vi "RobotDriveOpen6MotorWithTalonSRX.vi"(0 "Left Motor 1":u8=20, 1 "Left Motor 2":u8=20, 2 "Left Motor 3":u8=20, 3 "Right Motor 1":u8=20, 4 "Right Motor 2":u8=20, 5 "Right Motor 3":u8=20, 7 "error in (no error)":errorcluster, 8 "Left Motor Inverted 1":bool, 9 "Right Motor Inverted 1":bool, 10 "Left Motor Inverted 2":bool, 11 "Right Motor Inverted 2":bool, 12 "Left Motor Inverted 3":bool, 13 "Right Motor Inverted 3":bool) -> (20 "RobotDriveDevRef":T1={"DevStatus"={"status"=FALSE, "code"=0, "source"=""}, "Motors[]"=[], "Square Inputs"=FALSE, "Max Output"=1.0}, 27 "error out":errorcluster)   [LabVIEW 2015]
doc: "Opens a reference to the robot drive for a four-motor robot using VictorSP motor controllers.\n\nThis software is licensed. Open the labview\\readme\\WPI Robotics Library Open Source License.txt file for more information."
uses:
  <vilib>/Rock Robotics/WPI/RobotDrive/WPI_RobotDriveDevRef.ctl
  <vilib>/Rock Robotics/WPI/MotorControl/WPI_MotorControlDeviceRef.ctl
  <vilib>/Rock Robotics/WPI/MotorControl/WPI_MotorControlType.ctl
  <vilib>/Rock Robotics/SystemInterfaces/DIO/FPGA_DIOPWMChannel.ctl
  <vilib>/Rock Robotics/WPI/PWM/WPI_PWMDeadband.ctl
  <vilib>/Rock Robotics/WPI/CAN/Jaguar/SubVIs/WPI_CANJaguar_ControlMode.ctl
  <vilib>/Rock Robotics/WPI/CAN/TalonSRX/WPI_CANTalonSRX_APIControlMode.ctl
  <vilib>/Rock Robotics/WPI/SafetyOutput/WPI_SafetyOutputConfigMenu.ctl
  <vilib>/Rock Robotics/WPI/MotorControl/WPI_MotorControlOpenCANTalonSRX.vi
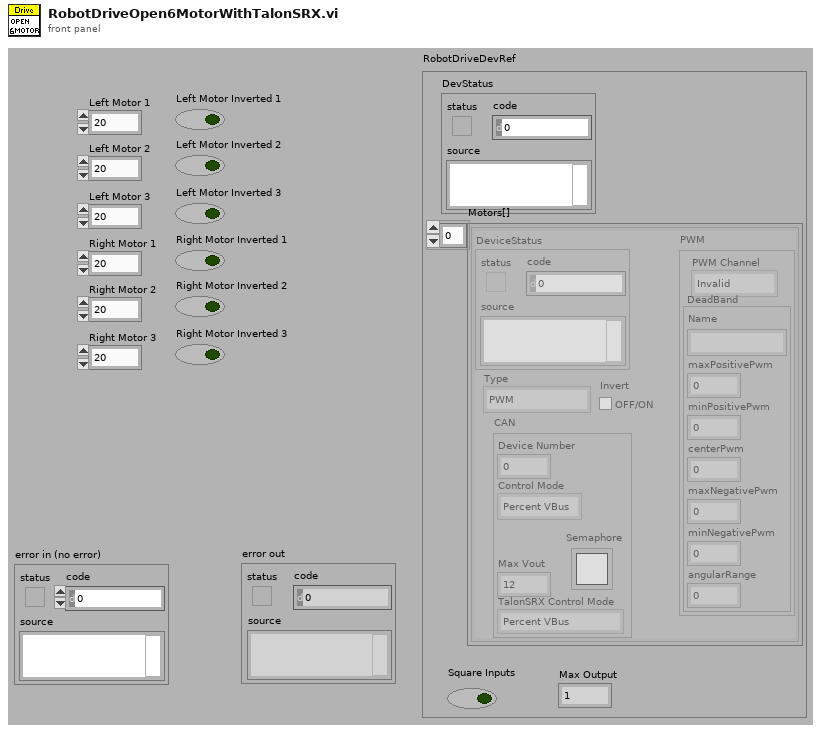
[diagram p1: front panel]
types:
  T1 = typedef "WPI_RobotDriveDevRef.ctl" = cluster{"DevStatus":errorcluster, "Motors[]":T2[], "Square Inputs":bool, "Max Output":dbl}
  T2 = typedef "WPI_MotorControlDeviceRef.ctl" = cluster{"DeviceStatus":errorcluster, "Type":T3, "PWM":cluster{"PWM Channel":T4, "DeadBand":T5}, "CAN":cluster{"Device Number":u8, "Control Mode":T6, "Semaphore":T7, "Max Vout":dbl, "TalonSRX Control Mode":T8}, "Invert":bool}
  T3 = typedef "WPI_MotorControlType.ctl" = enum16{"PWM", "CAN", "CANTalonSRX"}
  T4 = typedef "FPGA_DIOPWMChannel.ctl" = enum8{"PWM 0", "PWM 1", "PWM 2", "PWM 3", "PWM 4", "PWM 5", "PWM 6", "PWM 7", "PWM 8", "PWM 9", "PWM MXP 0", "PWM MXP 1", "PWM MXP 2", "PWM MXP 3", "PWM MXP 4", "PWM MXP 5", "PWM MXP 6", "PWM MXP 7", "PWM MXP 8", "PWM MXP 9", "Invalid"}
  T5 = typedef "WPI_PWMDeadband.ctl" = cluster{"Name":string, "maxPositivePwm":i32, "minPositivePwm":i32, "centerPwm":i32, "maxNegativePwm":i32, "minNegativePwm":i32, "angularRange":u16}
  T6 = typedef "WPI_CANJaguar_ControlMode.ctl" = enum8{"Percent VBus", "Current", "Speed", "Position", "Voltage"}
  T7 = typedef "Semaphore RefNum" = refnum<k1>
  T8 = typedef "WPI_CANTalonSRX_APIControlMode.ctl" = enum8{"Percent VBus", "Speed", "Position", "Slave", "Unchanged / Invalid", "Voltage Compensation", "Current", "Motion Profile"}
  T9 = typedef "WPI_SafetyOutputConfigMenu.ctl" = enum16{"Enable", "Disable"}
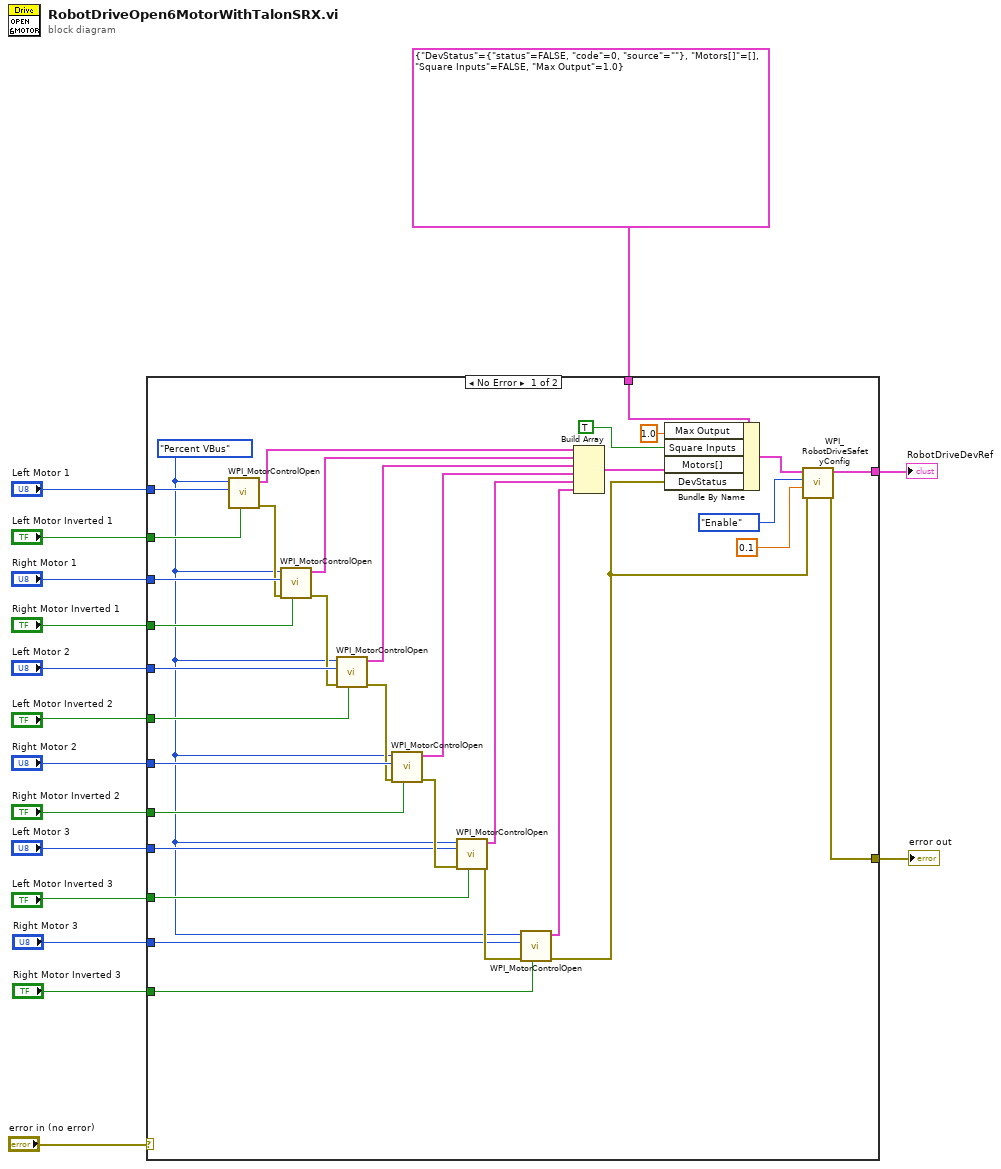
[diagram p0: block diagram]
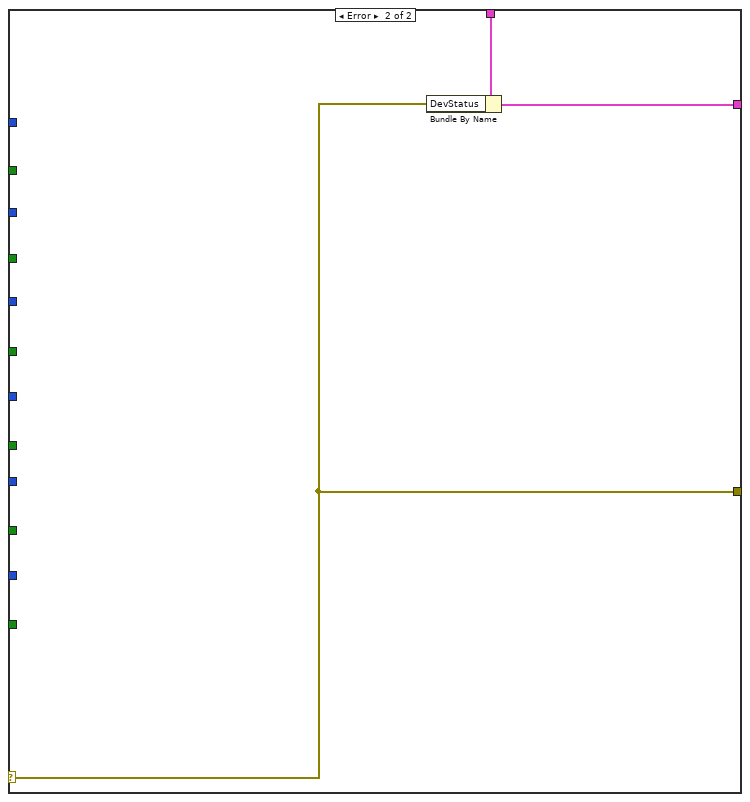
[diagram p2: hidden frame]
diagram:
  n1 = case shown="No Error" "error in (no error)" {
    selector: "error in (no error)" -> [_ w51]
    tunnel: [w29 w52] -> w16
    tunnel: T1 {"DevStatus"={"status"=FALSE, "code"=0, "source"=""}, "Motors[]"=[], "Square Inputs"=FALSE, "Max Output"=1.0} ("RobotDriveDevRef") -> [w50 w53]
    tunnel: "Left Motor 1" -> [w48 _]
    tunnel: "Right Motor 2" -> [w45 _]
    tunnel: "Left Motor 2" -> [w46 _]
    tunnel: "Right Motor 1" -> [w47 _]
    tunnel: "Left Motor Inverted 1" -> [w36 _]
    tunnel: "Right Motor Inverted 1" -> [w35 _]
    tunnel: "Right Motor Inverted 2" -> [w33 _]
    tunnel: "Left Motor Inverted 2" -> [w34 _]
    tunnel: [w30 w51] -> w5
    tunnel: "Left Motor 3" -> [w21 _]
    tunnel: "Left Motor Inverted 3" -> [w19 _]
    tunnel: "Right Motor 3" -> [w20 _]
    tunnel: "Right Motor Inverted 3" -> [w18 _]
    frame No Error {
      w17 = WPI_CANTalonSRX_APIControlMode."Percent VBus" ("Control Mode")
      n2 = call-poly <vilib>:"WPI_MotorControlOpen.vi"("Invert"=w36, "Device Number"=w48, "Control Mode"=w17) -> ("error out"=w38:errorcluster, "MotorControlDeviceRef"=w44:T2)  [unwired: 2 in, 5 out]
      n3 = call-poly <vilib>:"WPI_MotorControlOpen.vi"("Invert"=w35, "error in (no error)"=w38, "Device Number"=w47, "Control Mode"=w17) -> ("error out"=w39:errorcluster, "MotorControlDeviceRef"=w43:T2)  [unwired: 1 in, 5 out]
      n4 = call-poly <vilib>:"WPI_MotorControlOpen.vi"("Invert"=w34, "error in (no error)"=w39, "Device Number"=w46, "Control Mode"=w17) -> ("error out"=w40:errorcluster, "MotorControlDeviceRef"=w42:T2)  [unwired: 1 in, 5 out]
      n5 = call-poly <vilib>:"WPI_MotorControlOpen.vi"("Invert"=w33, "error in (no error)"=w40, "Device Number"=w45, "Control Mode"=w17) -> ("error out"=w26:errorcluster, "MotorControlDeviceRef"=w41:T2)  [unwired: 1 in, 5 out]
      n6 = call-poly <vilib>:"WPI_MotorControlOpen.vi"("Invert"=w19, "error in (no error)"=w26, "Device Number"=w21, "Control Mode"=w17) -> ("error out"=w25:errorcluster, "MotorControlDeviceRef"=w23:T2)  [unwired: 1 in, 5 out]
      n7 = call-poly <vilib>:"WPI_MotorControlOpen.vi"("Invert"=w18, "error in (no error)"=w25, "Device Number"=w20, "Control Mode"=w17) -> ("error out"=w24:errorcluster, "MotorControlDeviceRef"=w22:T2)  [unwired: 1 in, 5 out]
      n8 = Build Array(w44, w43, w42, w41, w23, w22) -> (w37:T2[])
      n9 = Bundle By Name(cluster=w50, "Max Output"=1.0, "Square Inputs"=TRUE ("DestroyPWM?"), "Motors[]"=w37, "DevStatus"=w24) -> (w31:T1)
      n10 = call <vilib>:"WPI_RobotDriveSafetyConfig.vi"("error in (no error)"=w24, "timeout (s)"=0.1, "mode"=WPI_SafetyOutputConfigMenu."Enable", "RobotDriveDevRef"=w31) -> ("error out"=w30:errorcluster, "RobotDriveDevRef"=w29:T1)  [unwired: 6 out]
    }
    frame Error {
      n11 = Bundle By Name(cluster=w53, "DevStatus"=w51) -> (w52:T1)
    }
  }
  "RobotDriveDevRef" <- w16
  "error out" <- w5
